vi "Directional Coupler.vi"() -> ()   [LabVIEW 2009]
uses:
  <vilib>/imath/engines/lvmath2/RunTimeEngine/ErrorHandling/NIMS_Finalize Error.vi
  <vilib>/imath/engines/lvmath2/RunTimeEngine/Parser/MC_Version.vi
  <vilib>/imath/engines/lvmath2/RunTimeEngine/Managers/WorkSpace/UID Generator.vi
  <vilib>/imath/engines/lvmath/Functions/Error Handling/error.ctl
  <vilib>/imath/engines/lvmath2/RunTimeEngine/NodeEndStatement/NIMS_NodeEndStatement_Output.vi
  <instcachedir>/0/NIMS_NodeEndStatement_Output_B70DDD75627E4997AAE11E9955EDAA25.lvgen/NIMS_NodeEndStatement_Output_B70DDD75627E4997AAE11E9955EDAA25_000.vi
  <vilib>/imath/engines/lvmath2/RunTimeEngine/Managers/SymbolTable/Clear UID.vi
  <vilib>/imath/engines/lvmath/Functions/Error Handling/MergeErrorsWrapper.vi
  <vilib>/imath/engines/lvmath2/RunTimeEngine/VariableToken/NIMS_VariableToken_CondDefined.vi
  <instcachedir>/0/NIMS_VariableToken_CondDefined_5641E79000FB4D628475532441475385.lvgen/NIMS_VariableToken_CondDefined_5641E79000FB4D628475532441475385_001.vi
  <vilib>/imath/engines/lvmath/Functions/Error Handling/MC_Mask_Errors.vi
  <vilib>/imath/engines/lvmath2/RunTimeEngine/BuiltInFunctions/rem/NIMS_rem_no checks.vi
  <instcachedir>/0/NIMS_rem_no checks_4CC9B305AB7E42EF90AFC4973FB32F8D.lvgen/NIMS_rem_no checks_4CC9B305AB7E42EF90AFC4973FB32F8D_000.vi
  <vilib>/imath/engines/lvmath2/RunTimeEngine/BuiltInFunctions/uint32/NIMS_uint32(real).vi
  <instcachedir>/0/NIMS_uint32(real)_FDC83D68D45943DDB8F3F934FF8A712F.lvgen/NIMS_uint32(real)_FDC83D68D45943DDB8F3F934FF8A712F_000.vi
  <vilib>/imath/engines/lvmath2/RunTimeEngine/BuiltInFunctions/double/NIMS_double.vi
  <instcachedir>/0/NIMS_double_2CE444F3CE4146B199A482FE12545E45.lvgen/NIMS_double_2CE444F3CE4146B199A482FE12545E45_000.vi
  <vilib>/imath/engines/lvmath2/RunTimeEngine/RangeToken/NIMS_Range.vi
  <instcachedir>/0/NIMS_Range_6D647EC16A744C98B5DE1D649A2D648D.lvgen/NIMS_Range_6D647EC16A744C98B5DE1D649A2D648D_001.vi
  <vilib>/imath/engines/lvmath2/RunTimeEngine/BuiltInFunctions/length/NIMS_length(GV).vi
  <instcachedir>/0/NIMS_length(GV)_7D6E94E728E145E68721C53861296D96.lvgen/NIMS_length(GV)_7D6E94E728E145E68721C53861296D96_000.vi
  <instcachedir>/0/NIMS_Range_6D647EC16A744C98B5DE1D649A2D648D.lvgen/NIMS_Range_6D647EC16A744C98B5DE1D649A2D648D_000.vi
  <vilib>/imathl/engines/lvmath/Functions/Error Handling/Create Error.vi
  <vilib>/imath/engines/lvmath2/RunTimeEngine/ReplaceToken/NIMS_Replace - V(S)=S.vi
  <instcachedir>/0/NIMS_Replace - V(S)=S_670A9E0533664C1D848C8E58B3321B6A.lvgen/NIMS_Replace - V(S)=S_670A9E0533664C1D848C8E58B3321B6A_002.vi
  <vilib>/imath/engines/lvmath2/RunTimeEngine/ReplaceToken/NIMS_Replace - Size Check _(_)=S.vi
  <instcachedir>/0/NIMS_Replace - Size Check _(_)=S_8596181D73404097BAB9CBB006194BB0.lvgen/NIMS_Replace - Size Check _(_)=S_8596181D73404097BAB9CBB006194BB0_002.vi
  <vilib>/imath/engines/lvmath2/RunTimeEngine/ReplaceToken/NIMS_Replace - Check Linear.vi
  <instcachedir>/0/NIMS_Replace - Check Linear_9243CBB174894FF6977027453DA6955E.lvgen/NIMS_Replace - Check Linear_9243CBB174894FF6977027453DA6955E_002.vi
  <vilib>/imath/engines/lvmath2/RunTimeEngine/VariableToken/NIMS_VariableToken_CondDefinedDefinedByReplace.vi
  <instcachedir>/0/NIMS_VariableToken_CondDefinedDefinedByReplace_D162CFFC24174562A9FEA619A91E1A56.lvgen/NIMS_VariableToken_CondDefinedDefinedByReplace_D162CFFC24174562A9FEA619A91E1A56_002.vi
  <vilib>/imath/engines/lvmath2/RunTimeEngine/CommandStatement/MC_CommandStatement_break.vi
  <vilib>/imath/engines/lvmath2/RunTimeEngine/LocalVariableDefStatement/MC_LocalVariableDefStatement_Display.vi
  <vilib>/imath/engines/lvmath2/RunTimeEngine/RunTimeType/NIMS_RunTimeType_From StrictType (excl LVString).vi
  <vilib>/imath/engines/lvmath2/RunTimeEngine/ArithmeticOperatorToken/NIMS_ArithmeticOperator_times.vi
  <instcachedir>/0/NIMS_ArithmeticOperator_times_3987BC660D7947CD8628C10658A43225.lvgen/NIMS_ArithmeticOperator_times_3987BC660D7947CD8628C10658A43225_001.vi
  <instcachedir>/0/NIMS_NodeEndStatement_Output_B70DDD75627E4997AAE11E9955EDAA25.lvgen/NIMS_NodeEndStatement_Output_B70DDD75627E4997AAE11E9955EDAA25_001.vi
  <instcachedir>/0/NIMS_ArithmeticOperator_times_3987BC660D7947CD8628C10658A43225.lvgen/NIMS_ArithmeticOperator_times_3987BC660D7947CD8628C10658A43225_000.vi
  <vilib>/imath/engines/lvmath2/RunTimeEngine/VariableToken/Read/NIMS_Get Elements - RV(_) - Check.vi
  <instcachedir>/0/NIMS_Get Elements - RV(_) - Check_60F12861D0564803969A5D0D0D1716CD.lvgen/NIMS_Get Elements - RV(_) - Check_60F12861D0564803969A5D0D0D1716CD_000.vi
  <vilib>/imath/engines/lvmath2/RunTimeEngine/BuiltInFunctions/abs/NIMS_abs(signed).vi
  <instcachedir>/0/NIMS_abs(signed)_C4FCB8E6058B49B797C7C8D53CA5F6EC.lvgen/NIMS_abs(signed)_C4FCB8E6058B49B797C7C8D53CA5F6EC_000.vi
  <vilib>/imath/engines/lvmath2/RunTimeEngine/BuiltInFunctions/cos/NIMS_cos(C).vi
  <instcachedir>/0/NIMS_cos(C)_0DF33C64BB6D4141A0AACB6BF03FEF51.lvgen/NIMS_cos(C)_0DF33C64BB6D4141A0AACB6BF03FEF51_000.vi
  <vilib>/imath/engines/lvmath2/RunTimeEngine/ArithmeticOperatorToken/NIMS_ArithmeticOperator_power(S).vi
  <instcachedir>/0/NIMS_ArithmeticOperator_power(S)_A502679C095F4520BDC53E297C98A9BD.lvgen/NIMS_ArithmeticOperator_power(S)_A502679C095F4520BDC53E297C98A9BD_002.vi
  <vilib>/imath/engines/lvmath2/RunTimeEngine/Managers/SymbolTable/NIMS_WorkSpace.lvlib
panel:
  in  "?":enum32{"DIRECTIONAL COUPLER"}(tab)
  out "ISOLATED PORT(Power dB)":dbl
  out "?":errorcluster
  in  "RADIUS OF THE HOLE(in mm)":dbl(slide) scale=1.6..2.5
  out "INPUT PORT(Power dB)":dbl
  out "THROUGH PORT(Power dB)":dbl
  out "COUPLED PORT(Power dB)":dbl
  out "COUPLING":dbl
  out "DIRECTIVITY":dbl
  out "ISOLATION":dbl
  in  "?":enum32{"ATTENUATOR"}(tab)
  out "?":dbl[](graph)
  in  "Set the value of attenuation in dB":dbl(slide) scale=0.0..100.0
  out "?":errorcluster
  in  "HELP FOR ATTENUATOR":bool
  out "error out":errorcluster
  in  "?":enum32{"ISOLATOR"}(tab)
  out "?":dbl[](graph)
  in  "?":bool
  out "?":errorcluster
  in  "HELP FOR ISOLATOR":bool
  out "error out":errorcluster
  in  "?":enum32{"MODULATOR"}(tab)
  out "?":dbl[](graph)
  in  "Modulating Frequency(KHz)":dbl(slide) scale=0.5..1.5
  out "?":errorcluster
  in  "HELP FOR MODULATOR":bool
  out "error out":errorcluster
  in  "?":enum32{"SOURCE"}(tab)
  out "?":dbl[](graph)
  in  "Frequency of carrier wave(GHz)":dbl(slide) scale=8.2..12.4
  in  "Voltage 3":dbl(knob) scale=0.0..20.0 scale format="%#_10g"
  out "?":errorcluster
  in  "HELP FOR SOURCE":bool
  out "error out":errorcluster
  # "VSWR meter"
  # "Source"
  # "Variable attenuator"
  # "Directional coupler"
  # "Coaxial to rectangular adapter"
  # "Connecting waveguide"
  # "Isolator"
  # "Connecting waveguide"
  # "Backward Direction"
  # "Forward direction"
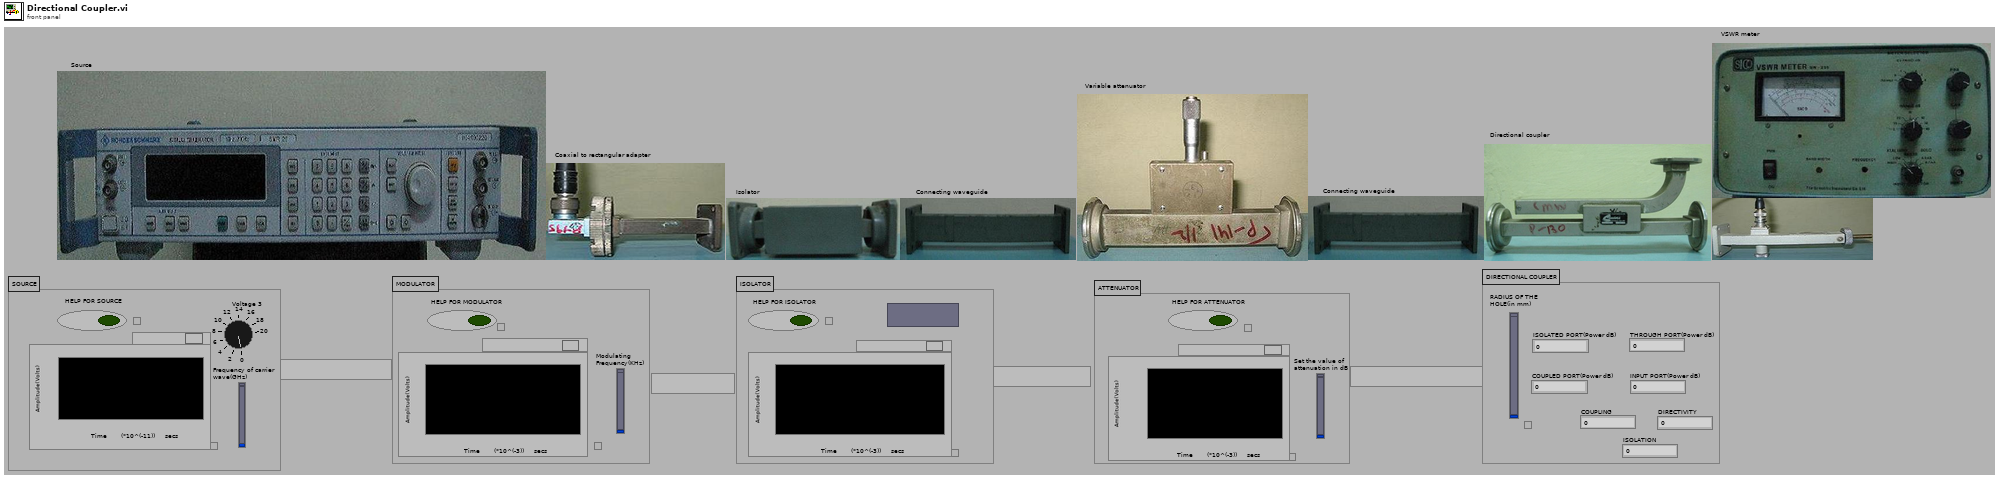
[diagram p1: front panel]
types:
  T1 = typedef "imagedata.ctl" = cluster{"image type":i32, "image depth":i32, "image":u8[], "mask":u8[], "colors":u32[], "Rectangle":cluster{"left":i16, "top":i16, "right":i16, "bottom":i16}}
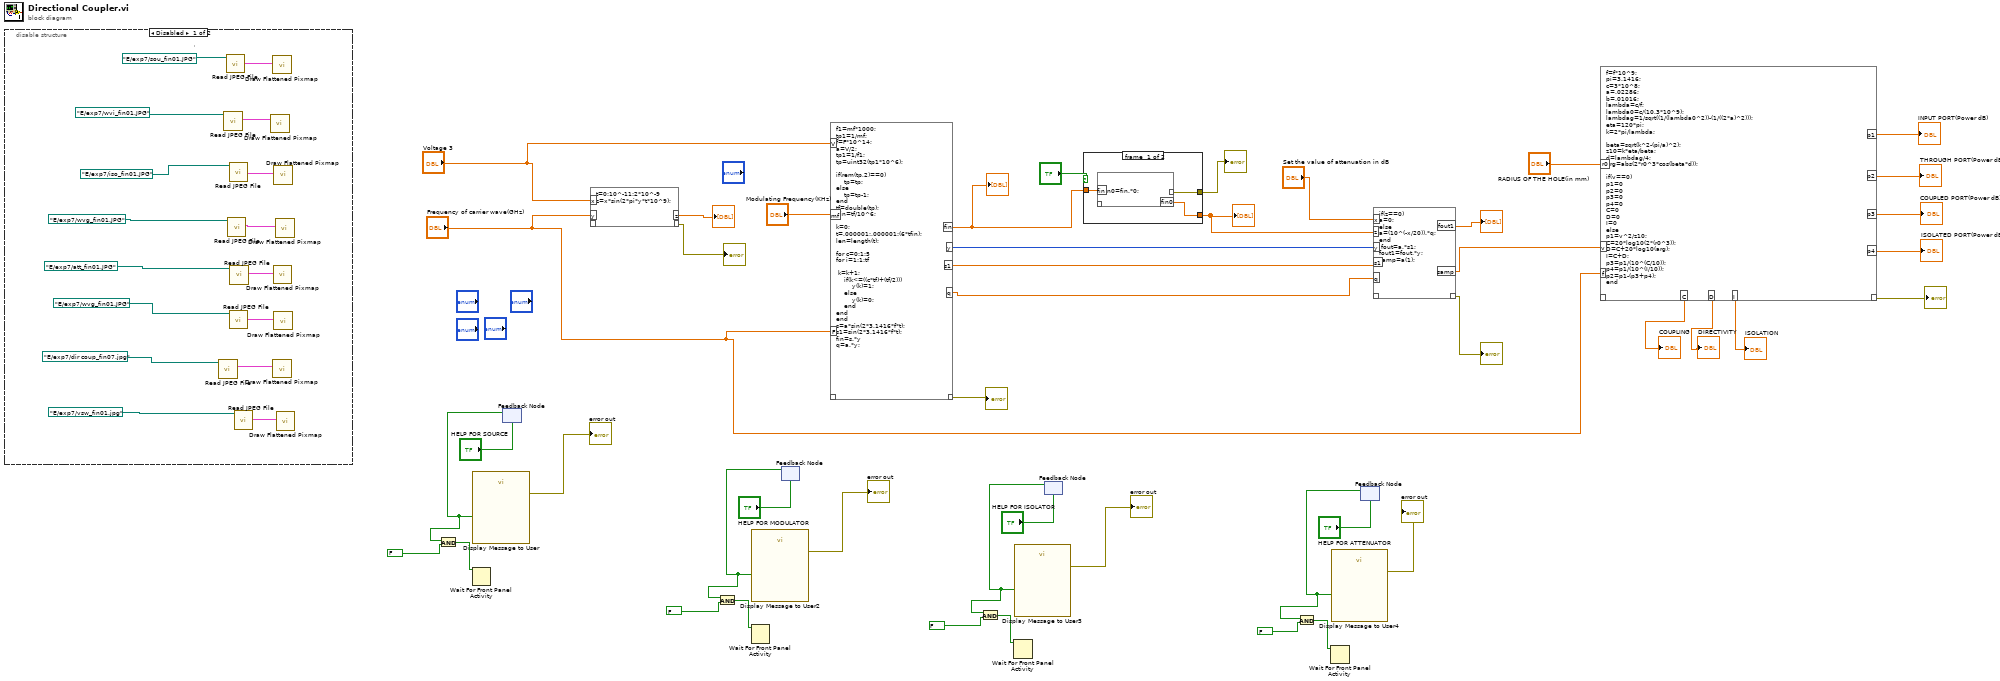
[diagram p0: block diagram]
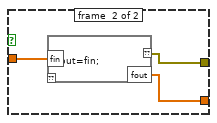
[diagram p3: hidden frame]
diagram:
  n1 = disable-structure shown="Disabled" {
    frame #0 {
      n2 = call <vilib>:"Read JPEG File.vi"("path to JPEG file"=path "E:/exp7/dir coup_fin07.jpg" ("Directional Coupler 2")) -> ("image data"=w52:T1)  [unwired: 8 in, 2 out]
      n3 = call <vilib>:"Read JPEG File.vi"("path to JPEG file"=path "E:/exp7/wvi_fin01.JPG" ("coaxial rectangular adapter")) -> ("image data"=w64:T1)  [unwired: 8 in, 2 out]
      n4 = call <vilib>:"Read JPEG File.vi"("path to JPEG file"=path "E:/exp7/sou_fin01.JPG" ("source")) -> ("image data"=w66:T1)  [unwired: 8 in, 2 out]
      n5 = call <vilib>:"Read JPEG File.vi"("path to JPEG file"=path "E:/exp7/wvg_fin01.JPG" ("Connecting waveguide")) -> ("image data"=w62:T1)  [unwired: 8 in, 2 out]
      n6 = call <vilib>:"Read JPEG File.vi"("path to JPEG file"=path "E:/exp7/iso_fin01.JPG" ("isolator")) -> ("image data"=w54:T1)  [unwired: 8 in, 2 out]
      n7 = call <vilib>:"Read JPEG File.vi"("path to JPEG file"=path "E:/exp7/wvg_fin01.JPG" ("Connecting Waveguide 3")) -> ("image data"=w59:T1)  [unwired: 8 in, 2 out]
      n8 = call <vilib>:"Read JPEG File.vi"("path to JPEG file"=path "E:/exp7/att_fin01.JPG" ("Variable Attenuator 2")) -> ("image data"=w53:T1)  [unwired: 8 in, 2 out]
      n9 = call <vilib>:"Read JPEG File.vi"("path to JPEG file"=path "E:/exp7/vsw_fin01.jpg" ("VSWR meter 2")) -> ("image data"=w55:T1)  [unwired: 8 in, 2 out]
      n10 = call <vilib>:"Draw Flattened Pixmap.vi"("image data"=w64) -> ()  [unwired: 8 in, 1 out]
      n11 = call <vilib>:"Draw Flattened Pixmap.vi"("image data"=w66) -> ()  [unwired: 8 in, 1 out]
      n12 = call <vilib>:"Draw Flattened Pixmap.vi"("image data"=w52) -> ()  [unwired: 8 in, 1 out]
      n13 = call <vilib>:"Draw Flattened Pixmap.vi"("image data"=w53) -> ()  [unwired: 8 in, 1 out]
      n14 = call <vilib>:"Draw Flattened Pixmap.vi"("image data"=w54) -> ()  [unwired: 8 in, 1 out]
      n15 = call <vilib>:"Draw Flattened Pixmap.vi"("image data"=w59) -> ()  [unwired: 8 in, 1 out]
      n16 = call <vilib>:"Draw Flattened Pixmap.vi"("image data"=w62) -> ()  [unwired: 8 in, 1 out]
      n17 = call <vilib>:"Draw Flattened Pixmap.vi"("image data"=w55) -> ()  [unwired: 8 in, 1 out]
    }
    frame #1 {
    }
  }
  n18 = feedback #1("HELP FOR SOURCE") -> (w21:bool)
  n19 = And(x=w21, y=FALSE) -> (x .and. y?=w19:bool)
  n20 = Wait For Front Panel Activity(3:w19) -> ()  [unwired: 3 out]
  n21 = call "Display Message to User"("Enable"=w21) -> ("error out"=→"error out":errorcluster, "CLOSE"=w23:bool)  [unwired: 2 in, 7 out]
  n22 = mathscript code="t=0:10^-11:2*10^-9\nz=x*sin(2*pi*y*t*10^9);"("x"="Voltage 3", "y"="Frequency of carrier wave(GHz)") -> ("??"=→"?":errorcluster, "z"=→"?":dbl[])  [unwired: 1 in]
  n23 = feedback #2("HELP FOR MODULATOR") -> (w15:bool)
  n24 = And(x=w15, y=FALSE) -> (x .and. y?=w13:bool)
  n25 = Wait For Front Panel Activity(3:w13) -> ()  [unwired: 3 out]
  n26 = call "Display Message to User2"("Enable"=w15) -> ("error out"=→"error out":errorcluster, "CLOSE"=w17:bool)  [unwired: 2 in, 7 out]
  n27 = mathscript code="f1=mf*1000;\ntp1=1/mf;\nf=F*10^14;\na=V/2;\ntp1=1/f1;\ntp=uint32(tp1*10^6);\n\nif(rem(tp,2)==0)\n    tp=tp;\nelse\n    tp=tp-1;\nend\ntf=double(tp);\ntfin=tf/10^6;\n\nk=0;\nt=.000001:.000001:(6*tfin);\nlen=length(t);\n\nfor c=0:1:5\nfor i=1:1:tf\n  \n k=k+1;\n    if(k<=((c*tf)+(tf/2)))\n        y(k)=1;\n    else\n        y(k)=0;\n    end\nend\nend\ns=a*sin(2*3.1416*f*t);\ns1=sin(2*3.1416*f*t);\nfin=s.*y\nq=a.*y;"("V"="Voltage 3", "mf"="Modulating Frequency(KHz)", "F"="Frequency of carrier wave(GHz)") -> ("??"=→"?":errorcluster, "y"=w29:i32[], "s1"=w33:dbl[], "q"=w25:dbl[], "fin"=w28:dbl[])  [unwired: 1 in]
  "?" <- w28
  n28 = feedback #3("HELP FOR ISOLATOR") -> (w9:bool)
  n29 = And(x=w9, y=FALSE) -> (x .and. y?=w7:bool)
  n30 = Wait For Front Panel Activity(3:w7) -> ()  [unwired: 3 out]
  n31 = call "Display Message to User3"("Enable"=w9) -> ("error out"=→"error out":errorcluster, "CLOSE"=w11:bool)  [unwired: 2 in, 7 out]
  n32 = case shown="True" "?" {
    tunnel: [w69 w90] -> w49
    tunnel: w28 -> [w67 w89]
    tunnel: [w68 w88] -> w26
    frame #0 {
      n33 = mathscript code="fin0=fin.*0;"("fin"=w67) -> ("??"=w69:errorcluster, "fin0"=w68:dbl[])  [unwired: 1 in]
    }
    frame #1 {
      n34 = mathscript code="fout=fin;"("fin"=w89) -> ("??"=w90:errorcluster, "fout"=w88:dbl[])  [unwired: 1 in]
    }
  }
  "?" <- w26
  "?" <- w49
  n35 = feedback #4("HELP FOR ATTENUATOR") -> (w3:bool)
  n36 = And(x=w3, y=FALSE) -> (x .and. y?=w1:bool)
  n37 = Wait For Front Panel Activity(3:w1) -> ()  [unwired: 3 out]
  n38 = call "Display Message to User4"("Enable"=w3) -> ("error out"=→"error out":errorcluster, "CLOSE"=w5:bool)  [unwired: 2 in, 7 out]
  n39 = mathscript code="if(z==0)\na=0; \nelse\na=(10^(-x/20)).*q;\nend\n fout=a.*s1;\nfout1=fout.*y;\nsamp=a(1);"("x"="Set the value of attenuation in dB", "z"=w26, "y"=w29, "s1"=w33, "q"=w25) -> ("??"=→"?":errorcluster, "fout1"=→"?":dbl[], "samp"=w32:dbl)  [unwired: 1 in]
  n40 = mathscript code="f=f*10^9;\npi=3.1416;\nc=3*10^8;\na=.02286;\nb=.01016;\nlambda=c/f;\nlambda0=c/(10.3*10^9);\nlambdag=1/sqrt((1/(lambda0^2))-(1/((2*a)^2)));\neta=120*pi;\nk=2*pi/lambda;\n\nbeta=sqrt(k^2-(pi/a)^2);\nz10=k*eta/beta;\nd=lambdag/4;\narg=abs(2*r0^3*cos(beta*d));\n\nif(v==0)\np1=0\np2=0\np3=0\np4=0\nC=0\nD=0\nI=0\nelse\np1=v^2/z10;\nC=20*log10(2*(r0^3));\nD=C+20*log10(arg);\nI=C+D;\np3=p1/(10^(C/10));\np4=p1/(10^(I/10));\np2=p1-(p3+p4);\nend"("v"=w32, "r0"="RADIUS OF THE HOLE(in mm)", "f"="Frequency of carrier wave(GHz)") -> ("??"=→"?":errorcluster, "p1"=→"INPUT PORT(Power dB)":dbl, "p2"=→"THROUGH PORT(Power dB)":dbl, "p3"=→"COUPLED PORT(Power dB)":dbl, "p4"=→"ISOLATED PORT(Power dB)":dbl, "C"=→"COUPLING":dbl, "D"=→"DIRECTIVITY":dbl, "I"=→"ISOLATION":dbl)  [unwired: 1 out]
